vi "NewConfigTable.vi"() -> ()   [LabVIEW 2011]
uses:
  <vilib>/Utility/file.llb/Write To Spreadsheet File (string).vi
panel:
  in  "Traverse Settings":string[][](table)
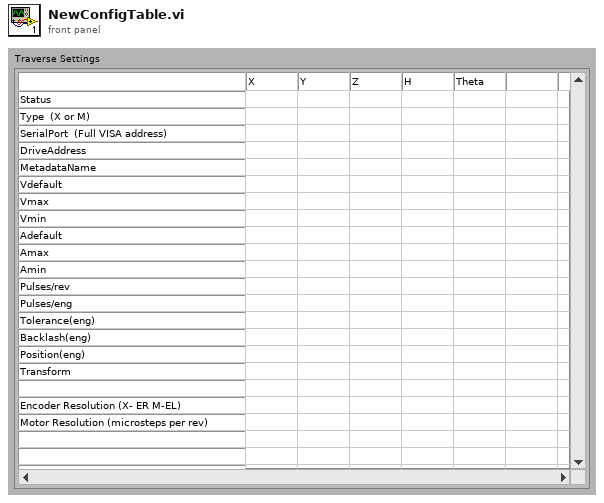
[diagram p1: front panel]
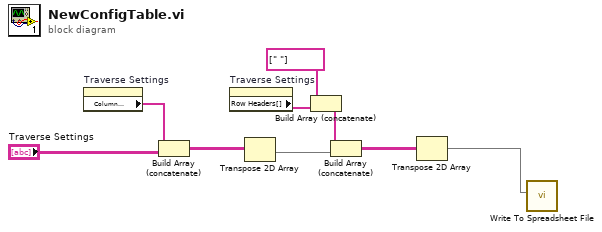
[diagram p0: block diagram]
diagram:
  n1 = property on="Traverse Settings" class="Tbl (strict)"() -> ("Column Headers[]"=w9:string[])  [unwired: 2 in, 2 out]
  n2 = Build Array (concatenate)(w9, "Traverse Settings") -> (w7:string[][])
  n3 = property on="Traverse Settings" class="Tbl (strict)"() -> ("Row Headers[]"=w4:string[])  [unwired: 2 in, 2 out]
  n4 = Transpose 2D Array(2D array=w7) -> (transposed array=w5:string[][])
  n5 = Build Array (concatenate)(string[] [" "], w4) -> (w2:string[])
  n6 = Build Array (concatenate)(w2, w5) -> (w6:string[][])
  n7 = Transpose 2D Array(2D array=w6) -> (transposed array=w1:string[][])
  n8 = call-poly <vilib>:"Write To Spreadsheet File.vi"("2D data"=w1) -> ()  [unwired: 7 in, 1 out]
